vi "niFpga wdp fft frame-based dummy.vi"(0 "real data in":fxp<+/-,8,1>[](array[numeric])=[0.0, 0.0], 5 "imaginary data in":fxp<+/-,8,1>[](array[numeric])=[0.0, 0.0], 9 "input frame start":bool, 12 "enable":bool) -> (3 "data indices":u16[](array[numeric]), 4 "real data out":fxp<+/-,19,12>[](array[numeric]), 6 "imaginary data out":fxp<+/-,19,12>[](array[numeric]), 10 "output valid":bool, 14 "ready for frame":bool, 15 "output frame start":bool)   [LabVIEW 2017]
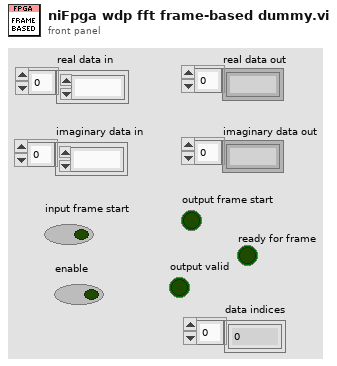
[diagram p1: front panel]
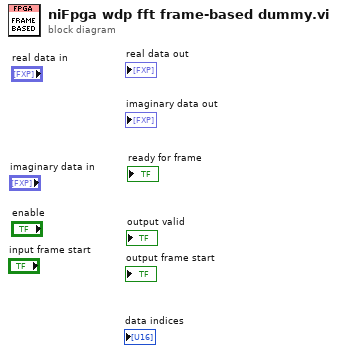
[diagram p0: block diagram]
diagram:
